vi "Goo01_F.vi"(11 "클러스터":T1={{"정지할 차이값"=0.08, "흰색과 밖 차이값"=0.15, "흰/검 반 값 "=0.3}, {"4: 오른각도"=122.0, "4: 뒷쪽각도"=0.0, "5: 오른각도"=120.0, "5: 앞쪽각도"=240.0, "6: 왼쪽각도"=250.0, "6: 앞쪽각도"=128.0}, {"2: 공각도"=233.0, "2: 굴릴각도"=60.0}}) -> (3 "ColorSensor":dbl[](array[numeric])=[2.440185297, 2.60009739, 2.598876687, 2.564697003])   [LabVIEW 2014]
uses:
  <vilib>/myRIO/Instrument Drivers/Onboard IO/AI/vis/Read.vi
  <vilib>/myRIO/Instrument Drivers/Onboard IO/AI/vis/Smart Open.vi
  <vilib>/Utility/error.llb/Error Cluster From Error Code.vi
  <vilib>/myRIO/Common/Instrument Driver Framework/myRIO v1.0/AI/vis/myRIO v1.0 Read AI.vi
panel:
  in  "앞 시간(ms)":u32=2300
  in  "스타트초":u32=1000
  in  "Select Servo":string(combo)="Servo 1"
  in  "1: 올리는 시간":u32=6000
  in  "1: 정지":u8=128
  in  "1: 올리기":u8=250
  out "2: 공각도":u8=233
  in  "Select Servo 6":string(combo)="Servo 6"
  in  "Select Servo 5":string(combo)="Servo 5"
  in  "Select Servo 4":string(combo)="Servo 4"
  in  "서브 컨트롤":u8=1
  # "시작할 때: 오른쪽 수평 맞추기"
  # "122"
  # "0"
  # "120"
  # "250"
  # "128"
  # "190"
  # "250"
  # "6000"
  # "128"
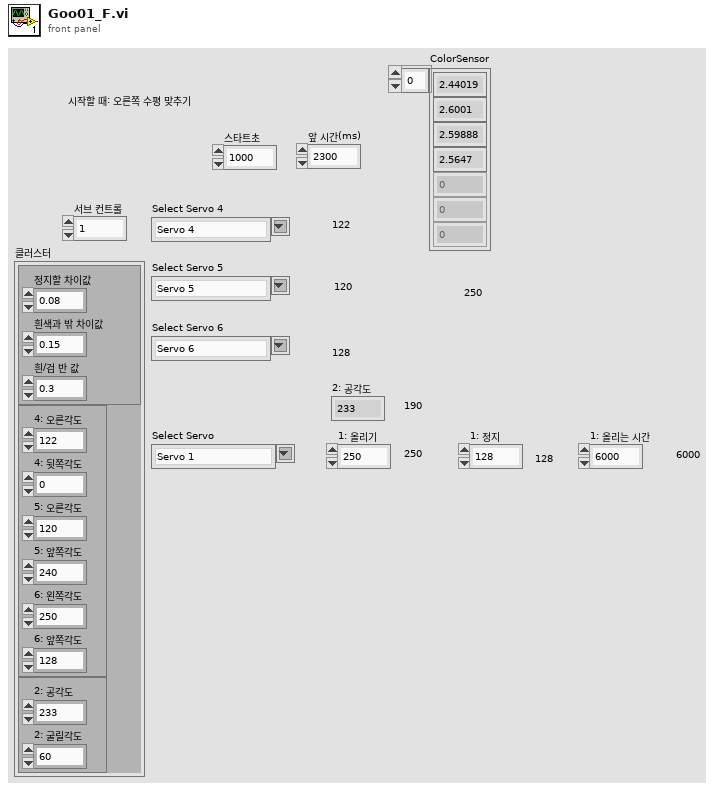
[diagram p1: front panel]
types:
  T1 = cluster{cluster{"정지할 차이값":dbl, "흰색과 밖 차이값":dbl, "흰/검 반 값 ":dbl}, cluster{"4: 오른각도":dbl, "4: 뒷쪽각도":dbl, "5: 오른각도":dbl, "5: 앞쪽각도":dbl, "6: 왼쪽각도":dbl, "6: 앞쪽각도":dbl}, cluster{"2: 공각도":dbl, "2: 굴릴각도":dbl}}
  T2 = cluster{"정지할 차이값":dbl, "흰색과 밖 차이값":dbl, "흰/검 반 값 ":dbl}
  T3 = cluster{"4: 오른각도":dbl, "4: 뒷쪽각도":dbl, "5: 오른각도":dbl, "5: 앞쪽각도":dbl, "6: 왼쪽각도":dbl, "6: 앞쪽각도":dbl}
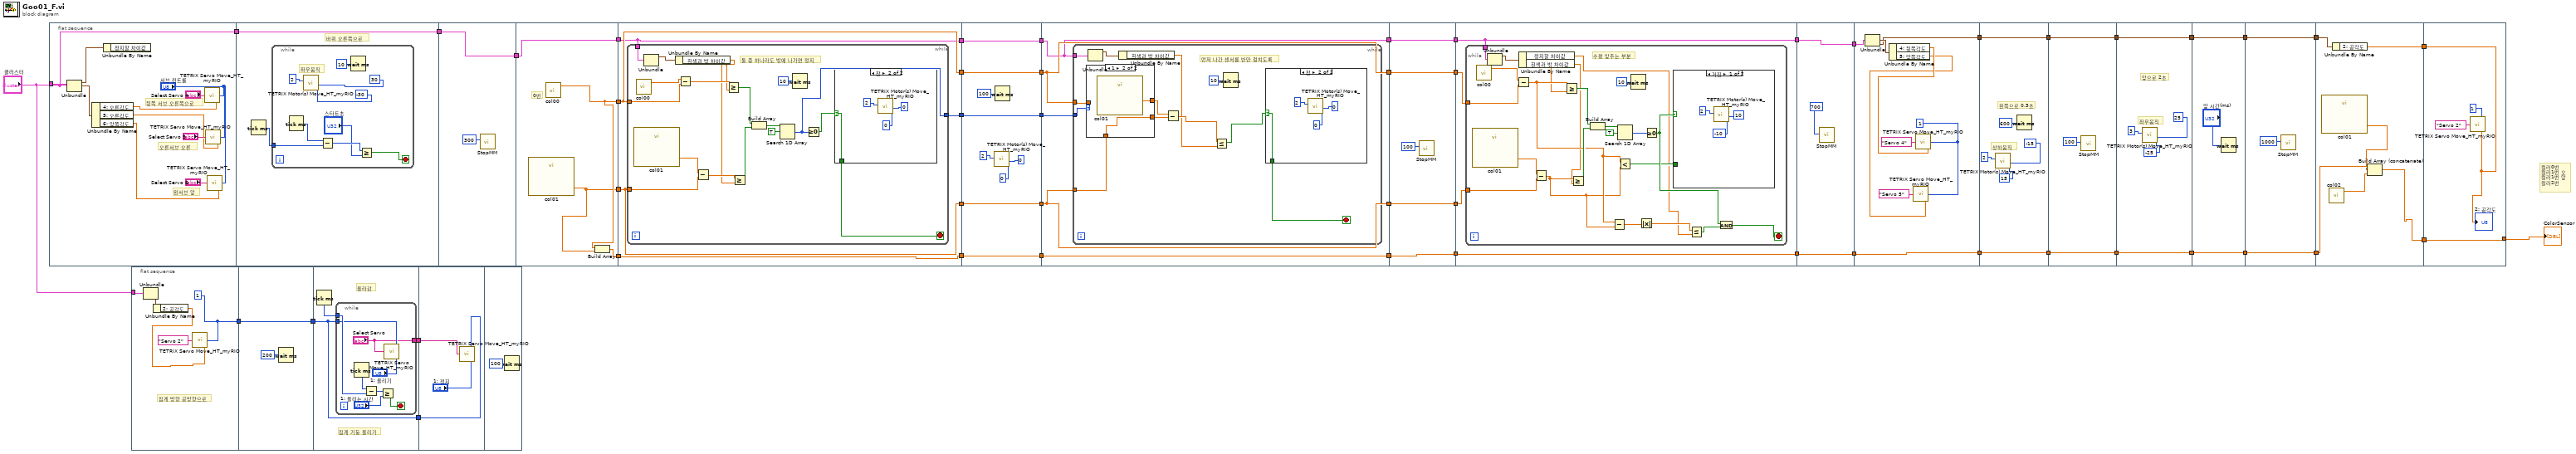
[diagram p0: block diagram]
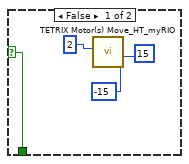
[diagram p2: hidden frame]
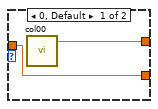
[diagram p3: hidden frame]
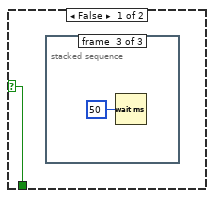
[diagram p4: hidden frame]
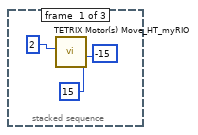
[diagram p5: hidden frame]
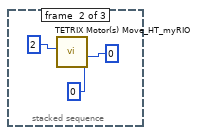
[diagram p6: hidden frame]
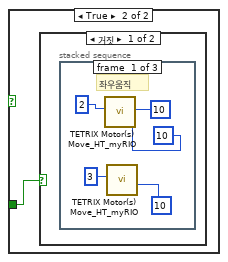
[diagram p7: hidden frame]
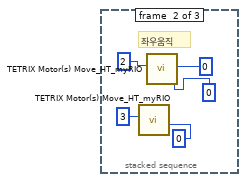
[diagram p8: hidden frame]
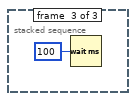
[diagram p9: hidden frame]
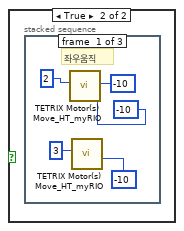
[diagram p10: hidden frame]
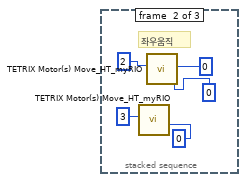
[diagram p11: hidden frame]
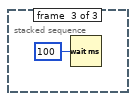
[diagram p12: hidden frame]
diagram:
  # "컬러0번\n컬러1번 오\n컬러1번 앞\n컬러2번"
  n1 = flat-sequence {
    tunnel: "클러스터" -> [w50]
    tunnel: [w50] -> w34
    tunnel: [w60] -> w35
    tunnel: w34 -> [w60]
    tunnel: [w71] -> w36
    tunnel: w35 -> [w71]
    tunnel: [w75] -> w49
    tunnel: [w74] -> w48
    tunnel: w36 -> [w76]
    tunnel: [w76] -> w33
    tunnel: [w73] -> w15
    tunnel: w49 -> [w80]
    tunnel: w48 -> [w81]
    tunnel: [w81] -> w47
    tunnel: [w80] -> w46
    tunnel: [w79] -> w38
    tunnel: w33 -> [w78]
    tunnel: [w78] -> w31
    tunnel: w15 -> [w77]
    tunnel: [w77] -> w12
    tunnel: w47 -> [w110]
    tunnel: w46 -> [w111]
    tunnel: [w111] -> w45
    tunnel: [w110] -> w44
    tunnel: [w109] -> w39
    tunnel: w38 -> [w109]
    tunnel: [w108] -> w32
    tunnel: w31 -> [w108]
    tunnel: [w107] -> w13
    tunnel: w12 -> [w107]
    tunnel: w45 -> [w120]
    tunnel: [w120] -> w43
    tunnel: w44 -> [w119]
    tunnel: [w119] -> w41
    tunnel: w39 -> [w118]
    tunnel: w32 -> [w117]
    tunnel: [w117] -> w29
    tunnel: [w116] -> w14
    tunnel: w13 -> [w116]
    tunnel: w43 -> [w153]
    tunnel: [w153] -> w42
    tunnel: w41 -> [w152]
    tunnel: [w152] -> w40
    tunnel: [w150] -> w30
    tunnel: w29 -> [w150]
    tunnel: w14 -> [w149]
    tunnel: [w149] -> w9
    tunnel: w42 -> [w157]
    tunnel: w40 -> [w156]
    tunnel: w30 -> [w155]
    tunnel: [w155] -> w27
    tunnel: [w154] -> w10
    tunnel: w9 -> [w154]
    tunnel: [w207] -> w28
    tunnel: w27 -> [w207]
    tunnel: [w206] -> w11
    tunnel: w10 -> [w206]
    tunnel: w28 -> [w217]
    tunnel: [w210] -> w21
    tunnel: w11 -> [w209]
    tunnel: [w209] -> w3
    tunnel: [w219] -> w22
    tunnel: w21 -> [w219]
    tunnel: [w218] -> w4
    tunnel: w3 -> [w218]
    tunnel: [w225] -> w23
    tunnel: w22 -> [w225]
    tunnel: [w224] -> w5
    tunnel: w4 -> [w224]
    tunnel: [w228] -> w24
    tunnel: w23 -> [w228]
    tunnel: [w227] -> w6
    tunnel: w5 -> [w227]
    tunnel: [w234] -> w25
    tunnel: w24 -> [w234]
    tunnel: [w233] -> w7
    tunnel: w6 -> [w233]
    tunnel: [w236] -> w26
    tunnel: w25 -> [w236]
    tunnel: [w235] -> w8
    tunnel: w7 -> [w235]
    tunnel: w26 -> [w243]
    tunnel: [w242] -> w20
    tunnel: w8 -> [w241]
    tunnel: [w238] -> w2
    tunnel: w20 -> [w247]
    tunnel: [w244] -> w1
    tunnel: w2 -> [w244]
    frame #0 {
      # "왼서브 앞"
      # "오른서브 오른"
      # "뒷쪽 서브 오른쪽으로"
      n2 = Unbundle(w50) -> (w51:T2, w55:T3)  [unwired: 1 out]
      n3 = Unbundle By Name(w55) -> ("4: 오른각도"=w54:dbl, "5: 오른각도"=w53:dbl, "6: 앞쪽각도"=w52:dbl)
      n4 = Unbundle By Name(w51) -> ()  [unwired: 1 out]
      n5 = call <vilib>:"TETRIX Servo Move_HT_myRIO.vi"("Servo Position (0 - 255)"=w54, "Controller Daisy Chain Position (1 - 4)"="서브 컨트롤", "Select Servo"="Select Servo 4") -> ()  [unwired: 2 in, 1 out]
      n6 = call <vilib>:"TETRIX Servo Move_HT_myRIO.vi"("Servo Position (0 - 255)"=w53, "Controller Daisy Chain Position (1 - 4)"="서브 컨트롤", "Select Servo"="Select Servo 5") -> ()  [unwired: 2 in, 1 out]
      n7 = call <vilib>:"TETRIX Servo Move_HT_myRIO.vi"("Servo Position (0 - 255)"=w52, "Controller Daisy Chain Position (1 - 4)"="서브 컨트롤", "Select Servo"="Select Servo 6") -> ()  [unwired: 2 in, 1 out]
    }
    frame #1 {
      # "바퀴 오른쪽으로"
      n8 = Tick Count (ms)() -> (millisecond timer value=w61:u32)
      n9 = while {
        tunnel: w61 -> [w66]
        stop <- w64 stop-if-true
        # "좌우움직"
        n10 = Tick Count (ms)() -> (millisecond timer value=w67:u32)
        n11 = call <vilib>:"TETRIX Motor(s) Move_HT_myRIO.vi"("Motor 2 Power (-100 to 100)\n0 = Stop/Brake\n-128 = Stop/Coast"=i8 -30 ("Motor 2 Power (-100 to 100)\n0 = Stop/Brake\n-128 = Stop/Coast"), "Motor 1 Power (-100 to 100)\n0 = Stop/Brake\n-128 = Stop/Coast"=i8 30 ("Motor 1 Power (-100 to 100)\n0 = Stop/Brake\n-128 = Stop/Coast"), "Controller Daisy Chain Position: 1 - 4"=u8 2) -> ()  [unwired: 6 in, 1 out]
        n12 = Subtract(x=w67, y=w66) -> (x-y=w65:u32)
        n13 = Wait (ms)(milliseconds to wait=u32 10 ("대기 시간(ms)")) -> ()  [unwired: 1 out]
        n14 = Greater Or Equal?(x=w65, y="스타트초") -> (x >= y?=w64:bool)
      }
    }
    frame #2 {
      n15 = call "StopMM.vi"("대기 시간(ms)"=u32 300) -> ()  [unwired: 11 in]
    }
    frame #3 {
      # "0번"
      n16 = call "col01.vi"() -> ("Col01 (B/AI1 (Pin 5))"=w74:dbl)  [unwired: 26 in, 1 out]
      n17 = call "col00.vi"() -> ("Col00 (B/AI0 (Pin 3))"=w75:dbl)  [unwired: 26 in, 1 out]
      n18 = Build Array(w75, w74) -> (w73:dbl[])
    }
    frame #4 {
      n19 = while {
        tunnel: w81 -> [w97]
        tunnel: w80 -> [w95]
        tunnel: [w86] -> w79
        tunnel: w78 -> [w85]
        stop <- w82 stop-if-true
        # "둘 중 하나라도 밖에 나가면 정지"
        n20 = call "col01.vi"() -> ("Col01 (B/AI1 (Pin 5))"=w98:dbl)  [unwired: 26 in, 1 out]
        n21 = call "col00.vi"() -> ("Col00 (B/AI0 (Pin 3))"=w96:dbl)  [unwired: 26 in, 1 out]
        n22 = Unbundle(w85) -> (w84:T2)  [unwired: 2 out]
        n23 = Unbundle By Name(w84) -> ("흰색과 밖 차이값"=w83:dbl)
        n24 = Subtract(x=w96, y=w95) -> (x-y=w94:dbl)
        n25 = Subtract(x=w98, y=w97) -> (x-y=w93:dbl)
        n26 = Greater Or Equal?(x=w94, y=w83) -> (x >= y?=w92:bool)
        n27 = Greater Or Equal?(x=w93, y=w83) -> (x >= y?=w91:bool)
        n28 = Build Array(w92, w91) -> (w90:bool[])
        n29 = Search 1D Array(1D array=w90, element=TRUE ("원소")) -> (index of element=w86:i32)  [unwired: 1 in]
        n30 = Wait (ms)(milliseconds to wait=u32 10 ("대기 시간(ms)")) -> ()  [unwired: 1 out]
        n31 = Greater Or Equal To 0?(x=w86) -> (x >= 0?=w87:bool)
        n32 = case shown="참" w87 {
          selector: w87 -> [w99 w103]
          tunnel: [w99 w103] -> w82
          frame False {
            n33 = call <vilib>:"TETRIX Motor(s) Move_HT_myRIO.vi"("Motor 2 Power (-100 to 100)\n0 = Stop/Brake\n-128 = Stop/Coast"=i8 -15 ("Motor 2 Power (-100 to 100)\n0 = Stop/Brake\n-128 = Stop/Coast"), "Motor 1 Power (-100 to 100)\n0 = Stop/Brake\n-128 = Stop/Coast"=i8 15 ("Motor 1 Power (-100 to 100)\n0 = Stop/Brake\n-128 = Stop/Coast"), "Controller Daisy Chain Position: 1 - 4"=u8 2) -> ()  [unwired: 6 in, 1 out]
          }
          frame True {
            n34 = call <vilib>:"TETRIX Motor(s) Move_HT_myRIO.vi"("Motor 2 Power (-100 to 100)\n0 = Stop/Brake\n-128 = Stop/Coast"=i8 0 ("Motor 2 Power (-100 to 100)\n0 = Stop/Brake\n-128 = Stop/Coast"), "Motor 1 Power (-100 to 100)\n0 = Stop/Brake\n-128 = Stop/Coast"=i8 0 ("Motor 1 Power (-100 to 100)\n0 = Stop/Brake\n-128 = Stop/Coast"), "Controller Daisy Chain Position: 1 - 4"=u8 2) -> ()  [unwired: 6 in, 1 out]
          }
        }
      }
    }
    frame #5 {
      n35 = call <vilib>:"TETRIX Motor(s) Move_HT_myRIO.vi"("Motor 2 Power (-100 to 100)\n0 = Stop/Brake\n-128 = Stop/Coast"=i8 0 ("Motor 2 Power (-100 to 100)\n0 = Stop/Brake\n-128 = Stop/Coast"), "Motor 1 Power (-100 to 100)\n0 = Stop/Brake\n-128 = Stop/Coast"=i8 0 ("Motor 1 Power (-100 to 100)\n0 = Stop/Brake\n-128 = Stop/Coast"), "Controller Daisy Chain Position: 1 - 4"=u8 2) -> ()  [unwired: 6 in, 1 out]
      n36 = Wait (ms)(milliseconds to wait=u32 100 ("대기 시간(ms)")) -> ()  [unwired: 1 out]
    }
    frame #6 {
      n37 = while {
        tunnel: w119 -> [w128]
        tunnel: w120 -> [w129]
        tunnel: w118 -> [w127]
        tunnel: w117 -> [w126]
        stop <- w124 stop-if-true
        # "먼저 나간 센서를 반만 걸치도록"
        n38 = case shown="1" w127 {
          tunnel: [w134 w135] -> w132
          tunnel: [w133 w136] -> w130
          tunnel: w129 -> [w133 _]
          tunnel: w128 -> [_ w136]
          frame 0, Default {
            n39 = call "col00.vi"() -> ("Col00 (B/AI0 (Pin 3))"=w134:dbl)  [unwired: 26 in, 1 out]
          }
          frame 1 {
            n40 = call "col01.vi"() -> ("Col01 (B/AI1 (Pin 5))"=w135:dbl)  [unwired: 26 in, 1 out]
          }
        }
        n41 = Unbundle(w126) -> (w125:T2)  [unwired: 2 out]
        n42 = Unbundle By Name(w125) -> ("흰색과 밖 차이값"=w121:dbl)
        n43 = Subtract(x=w132, y=w130) -> (x-y=w123:dbl)
        n44 = Less Or Equal?(x=w123, y=w121) -> (x <= y?=w122:bool)
        n45 = Wait (ms)(milliseconds to wait=u32 10 ("대기 시간(ms)")) -> ()  [unwired: 1 out]
        n46 = case shown="참" w122 {
          selector: w122 -> [w137 w145]
          tunnel: [w137 w145] -> w124
          frame False {
            n47 = stacked-sequence {
              frame #0 {
                n48 = call <vilib>:"TETRIX Motor(s) Move_HT_myRIO.vi"("Motor 2 Power (-100 to 100)\n0 = Stop/Brake\n-128 = Stop/Coast"=i8 15 ("Motor 2 Power (-100 to 100)\n0 = Stop/Brake\n-128 = Stop/Coast"), "Motor 1 Power (-100 to 100)\n0 = Stop/Brake\n-128 = Stop/Coast"=i8 -15 ("Motor 1 Power (-100 to 100)\n0 = Stop/Brake\n-128 = Stop/Coast"), "Controller Daisy Chain Position: 1 - 4"=u8 2) -> ()  [unwired: 6 in, 1 out]
              }
              frame #1 {
                n49 = call <vilib>:"TETRIX Motor(s) Move_HT_myRIO.vi"("Motor 2 Power (-100 to 100)\n0 = Stop/Brake\n-128 = Stop/Coast"=i8 0 ("Motor 2 Power (-100 to 100)\n0 = Stop/Brake\n-128 = Stop/Coast"), "Motor 1 Power (-100 to 100)\n0 = Stop/Brake\n-128 = Stop/Coast"=i8 0 ("Motor 1 Power (-100 to 100)\n0 = Stop/Brake\n-128 = Stop/Coast"), "Controller Daisy Chain Position: 1 - 4"=u8 2) -> ()  [unwired: 6 in, 1 out]
              }
              frame #2 {
                n50 = Wait (ms)(milliseconds to wait=u32 50 ("대기 시간(ms)")) -> ()  [unwired: 1 out]
              }
            }
          }
          frame True {
            n51 = call <vilib>:"TETRIX Motor(s) Move_HT_myRIO.vi"("Motor 2 Power (-100 to 100)\n0 = Stop/Brake\n-128 = Stop/Coast"=i8 0 ("Motor 2 Power (-100 to 100)\n0 = Stop/Brake\n-128 = Stop/Coast"), "Motor 1 Power (-100 to 100)\n0 = Stop/Brake\n-128 = Stop/Coast"=i8 0 ("Motor 1 Power (-100 to 100)\n0 = Stop/Brake\n-128 = Stop/Coast"), "Controller Daisy Chain Position: 1 - 4"=u8 2) -> ()  [unwired: 6 in, 1 out]
          }
        }
      }
    }
    frame #7 {
      n52 = call "StopMM.vi"("대기 시간(ms)"=u32 100) -> ()  [unwired: 11 in]
    }
    frame #8 {
      n53 = while {
        tunnel: w156 -> [w178]
        tunnel: w157 -> [w176]
        tunnel: w155 -> [w161]
        stop <- w169 stop-if-true
        # "수평 맞추는 부분"
        n54 = call "col01.vi"() -> ("Col01 (B/AI1 (Pin 5))"=w179:dbl)  [unwired: 26 in, 1 out]
        n55 = call "col00.vi"() -> ("Col00 (B/AI0 (Pin 3))"=w177:dbl)  [unwired: 26 in, 1 out]
        n56 = Unbundle(w161) -> (w160:T2)  [unwired: 2 out]
        n57 = Subtract(x=w177, y=w176) -> (x-y=w164:dbl)
        n58 = Unbundle By Name(w160) -> ("정지할 차이값"=w158:dbl, "흰색과 밖 차이값"=w159:dbl)
        n59 = Subtract(x=w179, y=w178) -> (x-y=w163:dbl)
        n60 = Greater Or Equal?(x=w164, y=w159) -> (x >= y?=w175:bool)
        n61 = Greater Or Equal?(x=w163, y=w159) -> (x >= y?=w174:bool)
        n62 = Build Array(w175, w174) -> (w173:bool[])
        n63 = Subtract(x=w164, y=w163) -> (x-y=w167:dbl)
        n64 = Search 1D Array(1D array=w173, element=TRUE ("원소")) -> (index of element=w171:i32)  [unwired: 1 in]
        n65 = Less?(x=w164, y=w163) -> (x < y?=w162:bool)
        n66 = Wait (ms)(milliseconds to wait=u32 10 ("대기 시간(ms)")) -> ()  [unwired: 1 out]
        n67 = Absolute Value(x=w167) -> (abs(x)=w166:dbl)
        n68 = Greater Or Equal To 0?(x=w171) -> (x >= 0?=w165:bool)
        n69 = case shown="거짓" w165 {
          tunnel: w162 -> [_ w183]
          frame False {
            n70 = call <vilib>:"TETRIX Motor(s) Move_HT_myRIO.vi"("Motor 2 Power (-100 to 100)\n0 = Stop/Brake\n-128 = Stop/Coast"=i8 -10 ("Motor 2 Power (-100 to 100)\n0 = Stop/Brake\n-128 = Stop/Coast"), "Motor 1 Power (-100 to 100)\n0 = Stop/Brake\n-128 = Stop/Coast"=i8 10 ("Motor 1 Power (-100 to 100)\n0 = Stop/Brake\n-128 = Stop/Coast"), "Controller Daisy Chain Position: 1 - 4"=u8 2) -> ()  [unwired: 6 in, 1 out]
          }
          frame True {
            n71 = case shown="거짓" w183 {
              frame False {
                n72 = stacked-sequence {
                  frame #0 {
                    # "좌우움직"
                    n73 = call <vilib>:"TETRIX Motor(s) Move_HT_myRIO.vi"("Motor 2 Power (-100 to 100)\n0 = Stop/Brake\n-128 = Stop/Coast"=i8 10 ("Motor 2 Power (-100 to 100)\n0 = Stop/Brake\n-128 = Stop/Coast"), "Motor 1 Power (-100 to 100)\n0 = Stop/Brake\n-128 = Stop/Coast"=i8 10 ("Motor 1 Power (-100 to 100)\n0 = Stop/Brake\n-128 = Stop/Coast"), "Controller Daisy Chain Position: 1 - 4"=u8 2) -> ()  [unwired: 6 in, 1 out]
                    n74 = call <vilib>:"TETRIX Motor(s) Move_HT_myRIO.vi"("Motor 1 Power (-100 to 100)\n0 = Stop/Brake\n-128 = Stop/Coast"=i8 10 ("Motor 1 Power (-100 to 100)\n0 = Stop/Brake\n-128 = Stop/Coast"), "Controller Daisy Chain Position: 1 - 4"=u8 3) -> ()  [unwired: 7 in, 1 out]
                  }
                  frame #1 {
                    # "좌우움직"
                    n75 = call <vilib>:"TETRIX Motor(s) Move_HT_myRIO.vi"("Motor 1 Power (-100 to 100)\n0 = Stop/Brake\n-128 = Stop/Coast"=i8 0 ("Motor 1 Power (-100 to 100)\n0 = Stop/Brake\n-128 = Stop/Coast"), "Controller Daisy Chain Position: 1 - 4"=u8 3) -> ()  [unwired: 7 in, 1 out]
                    n76 = call <vilib>:"TETRIX Motor(s) Move_HT_myRIO.vi"("Motor 2 Power (-100 to 100)\n0 = Stop/Brake\n-128 = Stop/Coast"=i8 0 ("Motor 2 Power (-100 to 100)\n0 = Stop/Brake\n-128 = Stop/Coast"), "Motor 1 Power (-100 to 100)\n0 = Stop/Brake\n-128 = Stop/Coast"=i8 0 ("Motor 1 Power (-100 to 100)\n0 = Stop/Brake\n-128 = Stop/Coast"), "Controller Daisy Chain Position: 1 - 4"=u8 2) -> ()  [unwired: 6 in, 1 out]
                  }
                  frame #2 {
                    n77 = Wait (ms)(milliseconds to wait=u32 100 ("대기 시간(ms)")) -> ()  [unwired: 1 out]
                  }
                }
              }
              frame True {
                n78 = stacked-sequence {
                  frame #0 {
                    # "좌우움직"
                    n79 = call <vilib>:"TETRIX Motor(s) Move_HT_myRIO.vi"("Motor 2 Power (-100 to 100)\n0 = Stop/Brake\n-128 = Stop/Coast"=i8 -10 ("Motor 2 Power (-100 to 100)\n0 = Stop/Brake\n-128 = Stop/Coast"), "Motor 1 Power (-100 to 100)\n0 = Stop/Brake\n-128 = Stop/Coast"=i8 -10 ("Motor 1 Power (-100 to 100)\n0 = Stop/Brake\n-128 = Stop/Coast"), "Controller Daisy Chain Position: 1 - 4"=u8 2) -> ()  [unwired: 6 in, 1 out]
                    n80 = call <vilib>:"TETRIX Motor(s) Move_HT_myRIO.vi"("Motor 1 Power (-100 to 100)\n0 = Stop/Brake\n-128 = Stop/Coast"=i8 -10 ("Motor 1 Power (-100 to 100)\n0 = Stop/Brake\n-128 = Stop/Coast"), "Controller Daisy Chain Position: 1 - 4"=u8 3) -> ()  [unwired: 7 in, 1 out]
                  }
                  frame #1 {
                    # "좌우움직"
                    n81 = call <vilib>:"TETRIX Motor(s) Move_HT_myRIO.vi"("Motor 1 Power (-100 to 100)\n0 = Stop/Brake\n-128 = Stop/Coast"=i8 0 ("Motor 1 Power (-100 to 100)\n0 = Stop/Brake\n-128 = Stop/Coast"), "Controller Daisy Chain Position: 1 - 4"=u8 3) -> ()  [unwired: 7 in, 1 out]
                    n82 = call <vilib>:"TETRIX Motor(s) Move_HT_myRIO.vi"("Motor 2 Power (-100 to 100)\n0 = Stop/Brake\n-128 = Stop/Coast"=i8 0 ("Motor 2 Power (-100 to 100)\n0 = Stop/Brake\n-128 = Stop/Coast"), "Motor 1 Power (-100 to 100)\n0 = Stop/Brake\n-128 = Stop/Coast"=i8 0 ("Motor 1 Power (-100 to 100)\n0 = Stop/Brake\n-128 = Stop/Coast"), "Controller Daisy Chain Position: 1 - 4"=u8 2) -> ()  [unwired: 6 in, 1 out]
                  }
                  frame #2 {
                    n83 = Wait (ms)(milliseconds to wait=u32 100 ("대기 시간(ms)")) -> ()  [unwired: 1 out]
                  }
                }
              }
            }
          }
        }
        n84 = Less Or Equal?(x=w166, y=w158) -> (x <= y?=w168:bool)
        n85 = And(x=w165, y=w168) -> (x .and. y?=w169:bool)
      }
    }
    frame #9 {
      n86 = call "StopMM.vi"("대기 시간(ms)"=u32 700) -> ()  [unwired: 11 in]
    }
    frame #10 {
      w213 = u8 1 ("Controller Daisy Chain Position (1 - 4)")
      n87 = Unbundle(w217) -> (w216:T3, w210:cluster{"2: 공각도":dbl, "2: 굴릴각도":dbl})  [unwired: 1 out]
      n88 = Unbundle By Name(w216) -> ("4: 뒷쪽각도"=w215:dbl, "5: 앞쪽각도"=w214:dbl)
      n89 = call <vilib>:"TETRIX Servo Move_HT_myRIO.vi"("Servo Position (0 - 255)"=w214, "Controller Daisy Chain Position (1 - 4)"=w213, "Select Servo"="Servo 5") -> ()  [unwired: 2 in, 1 out]
      n90 = call <vilib>:"TETRIX Servo Move_HT_myRIO.vi"("Servo Position (0 - 255)"=w215, "Controller Daisy Chain Position (1 - 4)"=w213, "Select Servo"="Servo 4") -> ()  [unwired: 2 in, 1 out]
    }
    frame #11 {
      # "왼쪽으로 0.5초"
      # "상하움직"
      n91 = call <vilib>:"TETRIX Motor(s) Move_HT_myRIO.vi"("Motor 2 Power (-100 to 100)\n0 = Stop/Brake\n-128 = Stop/Coast"=i8 15 ("Motor 2 Power (-100 to 100)\n0 = Stop/Brake\n-128 = Stop/Coast"), "Motor 1 Power (-100 to 100)\n0 = Stop/Brake\n-128 = Stop/Coast"=i8 -15 ("Motor 1 Power (-100 to 100)\n0 = Stop/Brake\n-128 = Stop/Coast"), "Controller Daisy Chain Position: 1 - 4"=u8 2) -> ()  [unwired: 6 in, 1 out]
      n92 = Wait (ms)(milliseconds to wait=u32 600 ("대기 시간(ms)")) -> ()  [unwired: 1 out]
    }
    frame #12 {
      n93 = call "StopMM.vi"("대기 시간(ms)"=u32 100) -> ()  [unwired: 11 in]
    }
    frame #13 {
      # "앞으로 2초"
      # "좌우움직"
      n94 = call <vilib>:"TETRIX Motor(s) Move_HT_myRIO.vi"("Motor 2 Power (-100 to 100)\n0 = Stop/Brake\n-128 = Stop/Coast"=i8 -25 ("Motor 2 Power (-100 to 100)\n0 = Stop/Brake\n-128 = Stop/Coast"), "Motor 1 Power (-100 to 100)\n0 = Stop/Brake\n-128 = Stop/Coast"=i8 25 ("Motor 1 Power (-100 to 100)\n0 = Stop/Brake\n-128 = Stop/Coast"), "Controller Daisy Chain Position: 1 - 4"=u8 3) -> ()  [unwired: 6 in, 1 out]
    }
    frame #14 {
      n95 = Wait (ms)(milliseconds to wait="앞 시간(ms)") -> ()  [unwired: 1 out]
    }
    frame #15 {
      n96 = call "StopMM.vi"("대기 시간(ms)"=u32 1000) -> ()  [unwired: 11 in]
    }
    frame #16 {
      n97 = call "col01.vi"() -> ("Col01 (B/AI1 (Pin 5))"=w240:dbl)  [unwired: 26 in, 1 out]
      n98 = call "col02.vi"() -> ("Col02 (B/AI2 (Pin 7))"=w239:dbl)  [unwired: 26 in, 1 out]
      n99 = Unbundle By Name(w243) -> ("2: 공각도"=w242:dbl)
      n100 = Build Array (concatenate)(w241, w240, w239) -> (w238:dbl[])
    }
    frame #17 {
      n101 = call <vilib>:"TETRIX Servo Move_HT_myRIO.vi"("Servo Position (0 - 255)"=w247, "Controller Daisy Chain Position (1 - 4)"=u8 1, "Select Servo"="Servo 2") -> ()  [unwired: 2 in, 1 out]
      "2: 공각도" <- w247
    }
  }
  n102 = flat-sequence {
    tunnel: "클러스터" -> [w251]
    tunnel: [w248] -> w18
    tunnel: [w253] -> w19
    tunnel: w18 -> [w253]
    tunnel: w19 -> [w256]
    tunnel: [w256] -> w17
    tunnel: [w255] -> w16
    tunnel: w17 -> [w267]
    tunnel: w16 -> [w266]
    frame #0 {
      w248 = u8 1 ("Controller Daisy Chain Position (1 - 4)")
      # "집게 방향 공방향으로"
      n103 = Unbundle(w251) -> (w250:cluster{"2: 공각도":dbl, "2: 굴릴각도":dbl})  [unwired: 2 out]
      n104 = Unbundle By Name(w250) -> ("2: 공각도"=w249:dbl)
      n105 = call <vilib>:"TETRIX Servo Move_HT_myRIO.vi"("Servo Position (0 - 255)"=w249, "Controller Daisy Chain Position (1 - 4)"=w248, "Select Servo"="Servo 2") -> ()  [unwired: 2 in, 1 out]
    }
    frame #1 {
      n106 = Wait (ms)(milliseconds to wait=u32 200 ("대기 시간(ms)")) -> ()  [unwired: 1 out]
    }
    frame #2 {
      # "집게 기둥 올리기"
      # "올라감"
      n107 = Tick Count (ms)() -> (millisecond timer value=w257:u32)
      n108 = while {
        tunnel: w257 -> [w264]
        tunnel: w256 -> [w259]
        tunnel: ["Select Servo"] -> w255
        stop <- w262 stop-if-true
        n109 = Tick Count (ms)() -> (millisecond timer value=w265:u32)
        n110 = Subtract(x=w265, y=w264) -> (x-y=w263:u32)
        n111 = Greater Or Equal?(x=w263, y="1: 올리는 시간") -> (x >= y?=w262:bool)
        n112 = call <vilib>:"TETRIX Servo Move_HT_myRIO.vi"("Servo Position (0 - 255)"="1: 올리기", "Controller Daisy Chain Position (1 - 4)"=w259, "Select Servo"="Select Servo") -> ()  [unwired: 2 in, 1 out]
      }
    }
    frame #3 {
      n113 = call <vilib>:"TETRIX Servo Move_HT_myRIO.vi"("Servo Position (0 - 255)"="1: 정지", "Controller Daisy Chain Position (1 - 4)"=w267, "Select Servo"=w266) -> ()  [unwired: 2 in, 1 out]
    }
    frame #4 {
      n114 = Wait (ms)(milliseconds to wait=u32 100 ("대기 시간(ms)")) -> ()  [unwired: 1 out]
    }
  }
  "ColorSensor" <- w1
